vi "UDP_Client.vi"() -> ()   [LabVIEW 2020]
uses:
  f190c7a5-feb0-4201-9828-7853bc1d3dd9.vi
panel:
  out "Read":string
  in  "LED On":bool
  in  "IP":string="192.168.85.175"
  out "Error Out":errorcluster
  in  "Stop":bool
  out "Time":u32
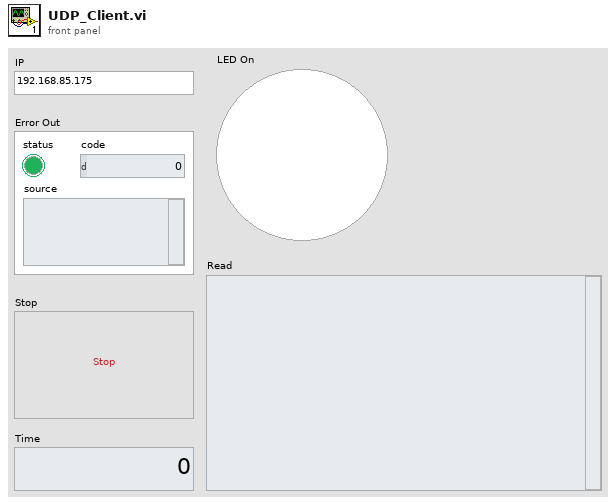
[diagram p1: front panel]
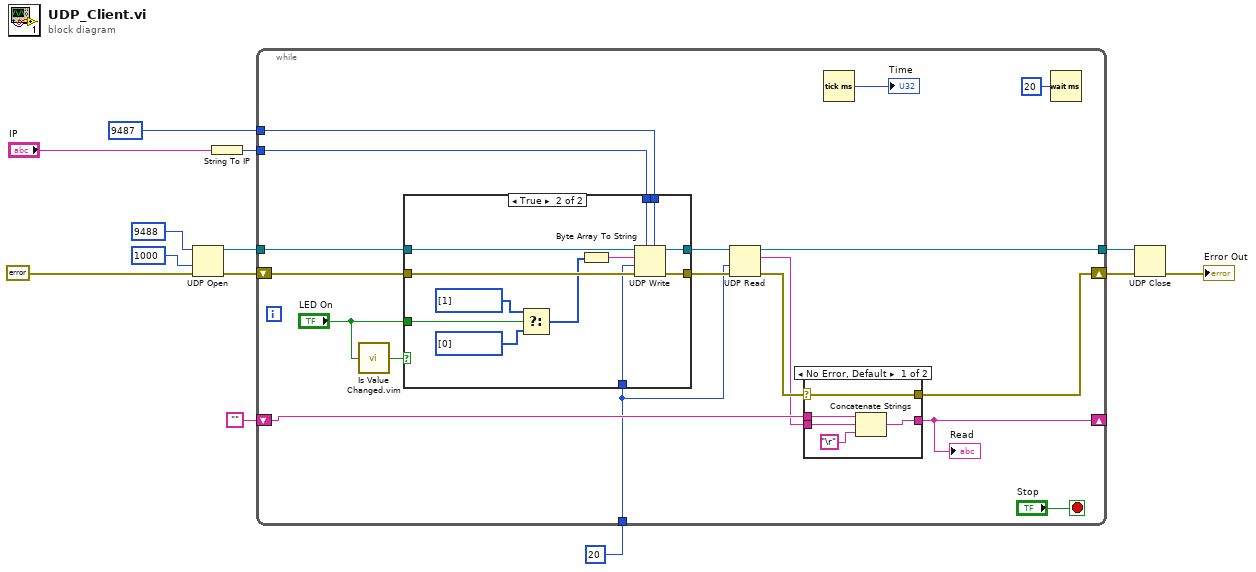
[diagram p0: block diagram]
diagram:
  n1 = UDP Open(8:errorcluster {"status"=FALSE, "code"=0, "source"=""} ("error in (no error)"), 9:1000 ("timeout ms (25000)"), 11:u16 9488 ("port")) -> (port=w9:refnum<k16>, 0:w12:errorcluster)  [unwired: 2 in, 1 out]
  n2 = String To IP(1:"IP") -> (0:w8:u32)
  n3 = while {
    shift-right: [w15] -> w3
    shift-left: w12 -> [w30]
    tunnel: w9 -> [w29]
    tunnel: w8 -> [w28]
    tunnel: u16 9487 ("port or service name") -> [w27]
    tunnel: [w19] -> w5
    shift-right: [w14] -> _
    shift-left: "" -> [w18]
    tunnel: 20 ("timeout ms (25000)") -> [w16]
    stop <- "Stop" stop-if-true
    n4 = call "Is Value Changed.vim"("value"="LED On") -> ("changed or first call?"=w22:bool)
    n5 = case shown="True" w22 {
      tunnel: w30 -> [w39 w51]
      tunnel: w29 -> [w38 w50]
      tunnel: w28 -> [_ w49]
      tunnel: w27 -> [_ w48]
      tunnel: [w39 w47] -> w21
      tunnel: [w38 w46] -> w20
      tunnel: "LED On" -> [_ w45]
      tunnel: w16 -> [_ w40]
      frame False {
      }
      frame True {
        n6 = Select(t=u8[] [1], s=w45, f=u8[] [0]) -> (s? t:f=w42:u8[])
        n7 = Byte Array To String(unsigned byte array=w42) -> (string=w41:string)
        n8 = UDP Write(address=w49, port or service name=w48, connection ID=w50, data in=w41, 8:w51, 9:w40) -> (error out=w47:errorcluster, 3:w46:refnum<k16>)
      }
    }
    n9 = UDP Read(connection ID=w20, timeout ms (25000)=w16, 8:w21) -> (data out=w17:string, error out=w31:errorcluster, 3:w19:refnum<k16>)  [unwired: 1 in, 2 out]
    n10 = case shown="No Error, Default" w31 {
      selector: w31 -> [w32 _]
      tunnel: w18 -> [w36 w37]
      tunnel: w17 -> [w35 _]
      tunnel: [w34 w37] -> w14
      tunnel: [w32 _] -> w15
      frame No Error {
        n11 = Concatenate Strings(w36, w35, "\r") -> (w34:string)
      }
      frame Error {
      }
    }
    "Read" <- w14
    n12 = Tick Count (ms)() -> (millisecond timer value=→"Time":u32)
    n13 = Wait (ms)(milliseconds to wait=u32 20) -> ()  [unwired: 1 out]
  }
  n14 = UDP Close(connection ID=w5, 8:w3) -> (error out=→"Error Out":errorcluster)  [unwired: 1 out]
